vi "compileAndRunScript.vi"(6 "data":variant, 8 "error in (no error)":errorcluster, 9 "CompiledList":refnum<class "CompiledList.lvclass">, 10 "HWControllerEvents in":refnum<class "HWControllerEvents.lvclass">, 11 "Compiler in":refnum<class "Compiler.lvclass">) -> (0 "error out":errorcluster, 3 "Compiler out":refnum<class "Compiler.lvclass">)   [LabVIEW 2011, in "Compiler.lvlib" / "Compiler.lvclass"]
uses:
  Compiler.lvclass
  CompiledList/CompiledList.lvclass
  Hal/HWController/HWControllerEvents/HWControllerEvents.lvclass
  Compiler.lvclass/Compiler.ctl
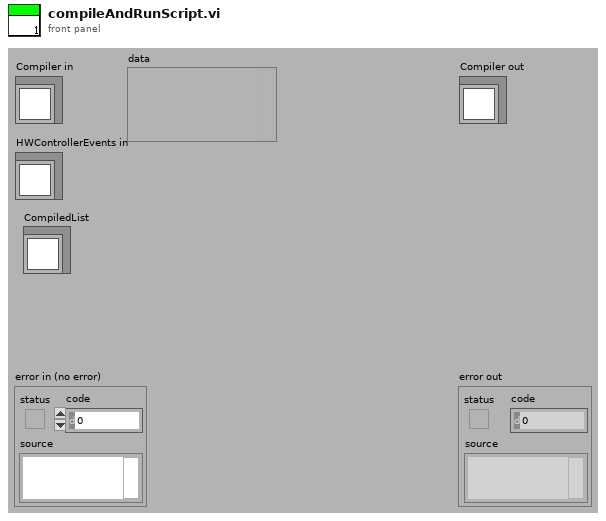
[diagram p1: front panel]
types:
  T1 = enum16{"start", "stop", "statusInquiry", "configure", "resetError", "resourcesInquiry", "reserveResources", "initialise", "resetAllChannels", "staticUpdate", "close", "HWStatus", "error", "resourcesAvailable", "resourcesReserved", "compilerError", "compiledScript", "compilingScript", "runScript", "configureCompiledScript"}
  T2 = cluster{"incomingEventTypes":cluster{"start":cluster{"Boolean":bool}, "stop":cluster{"Boolean":bool}, "statusInquiry":cluster{"Boolean":bool}, "configure":cluster{"DPScriptPath":path, "TimeStamp":string, "HWLoop?":bool}, "resetError":cluster{"Boolean":bool}, "resourcesInquiry":cluster{"Boolean":bool}, "reserveResources":cluster{"HWList":string[]}, "initialise":cluster{"HWList":string[]}, "close":cluster{"Boolean":bool}, "resetAllChannels":cluster{"Boolean":bool}, "staticChannelUpdate":cluster{"channel_address":string, "calibratedValue":dbl}, "runScript":cluster{"DPScriptPath":path, "TimeStamp":string, "HWLoop?":bool}, "compilingScript":cluster{"Path":path}, "compiledScript":cluster{"Path":path, "timeCompileAt":string}, "compilerError":cluster{"Path":path}, "configureCompiledScript":cluster{"DPScriptPath":path, "TimeStamp":string, "HWLoop?":bool, "CompiledScript":cluster{"ScriptListCompiler.lvclass":refnum<class "ScriptListCompiler.lvclass">, "aoChannels":refnum<class "AnalogOutput.lvclass">[], "doChannels":refnum<class "DigitalOutput.lvclass">[], "rfChannels":refnum<class "DDSOutput.lvclass">[]}}, "restartCompiler":cluster{"restart":bool}, "staticRfChannelUpdate":cluster{"channel_address":string, "Output":cluster{"Frequency(MHz)":dbl, "Amplitude":dbl, "Phase":dbl, "OutputForm":enum16{"Sine", "Square", "Triangle", "Arbitrary"}}}, "cameraUpdate":cluster{"Camera":string, "Type":string, "settings":path}}, "outgoingEventTypes":cluster{"HWStatus":cluster{"status":enum16{"Ready", "Compiling", "Configured", "Running", "Stopping", "Unresolved Error"}}, "error":cluster{"error out":errorcluster}, "resourcesAvailable":cluster{"availableHWList":string[], "reservedHWList":string[]}, "resourcesReserved":cluster{"reservedHWList":string[]}}}
  T3 = cluster{"DPScriptPath":path, "TimeStamp":string, "HWLoop?":bool, "CompiledScript":cluster{"ScriptListCompiler.lvclass":refnum<class "ScriptListCompiler.lvclass">, "aoChannels":refnum<class "AnalogOutput.lvclass">[], "doChannels":refnum<class "DigitalOutput.lvclass">[], "rfChannels":refnum<class "DDSOutput.lvclass">[]}}
  T4 = cluster{"DPScriptPath":path, "TimeStamp":string, "HWLoop?":bool}
  T5 = cluster{"ScriptListCompiler.lvclass":refnum<class "ScriptListCompiler.lvclass">, "aoChannels":refnum<class "AnalogOutput.lvclass">[], "doChannels":refnum<class "DigitalOutput.lvclass">[], "rfChannels":refnum<class "DDSOutput.lvclass">[]}
  T6 = cluster{"eventId":enum16{"start", "stop", "statusInquiry", "configure", "resetError", "resourcesInquiry", "reserveResources", "initialise", "resetAllChannels", "staticUpdate", "close", "HWStatus", "error", "resourcesAvailable", "resourcesReserved", "compilerError", "compiledScript", "compilingScript", "runScript", "configureCompiledScript"}, "configureCompiledScript":cluster{"DPScriptPath":path, "TimeStamp":string, "HWLoop?":bool, "CompiledScript":cluster{"ScriptListCompiler.lvclass":refnum<class "ScriptListCompiler.lvclass">, "aoChannels":refnum<class "AnalogOutput.lvclass">[], "doChannels":refnum<class "DigitalOutput.lvclass">[], "rfChannels":refnum<class "DDSOutput.lvclass">[]}}}
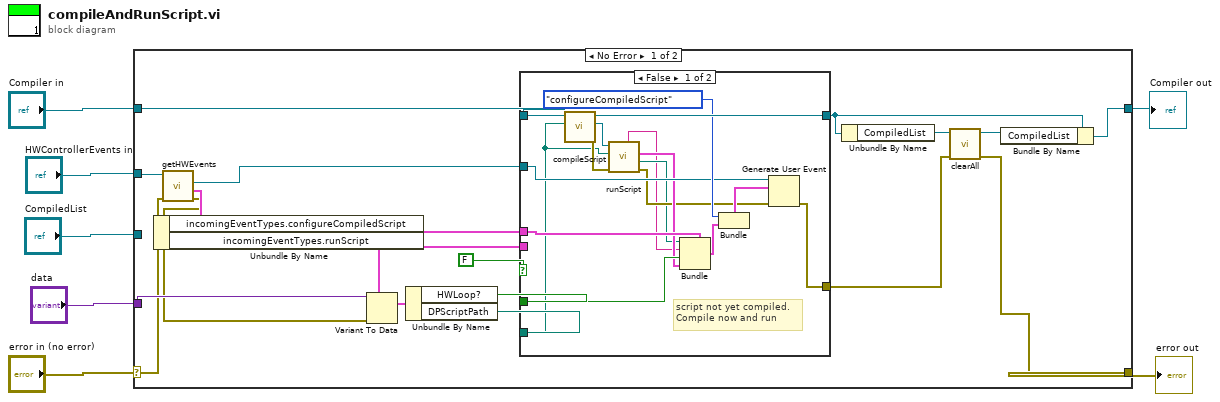
[diagram p0: block diagram]
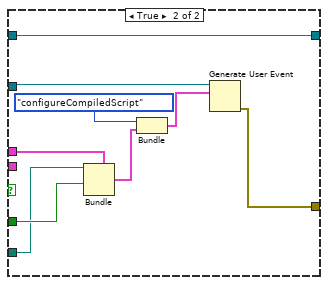
[diagram p2: hidden frame]
diagram:
  n1 = case shown="No Error" "error in (no error)" {
    selector: "error in (no error)" -> [w18 w53]
    tunnel: [w8 w53] -> w1
    tunnel: [w11 w52] -> w2
    tunnel: "Compiler in" -> [w16 w52]
    tunnel: "HWControllerEvents in" -> [w26 _]
    tunnel: "CompiledList" -> [_ _]
    tunnel: "data" -> [w24 _]
    frame No Error {
      n2 = call-dynamic "getHWEvents.vi"("error in (no error)"=w18, "HWControllerEvents in"=w26) -> ("error out"=w17:errorcluster, "eventDataTypes"=w25:T2, "HWCEvent"=w21:refnum<user-event>)  [unwired: 6 in, 1 out]
      n3 = Unbundle By Name(w25) -> ("incomingEventTypes.configureCompiledScript"=w20:T3, "incomingEventTypes.runScript"=w19:T4)
      n4 = Variant To Data(error in=w17, type=w19, Variant=w24) -> (data=w23:T4)  [unwired: 1 out]
      n5 = Unbundle By Name(w23) -> ("HWLoop?"=w22:bool, "DPScriptPath"=w15:path)
      n6 = case shown="False" FALSE {
        tunnel: [w41 w51] -> w12
        tunnel: w16 -> [w42 w51]
        tunnel: w22 -> [w36 w49]
        tunnel: w21 -> [w34 w48]
        tunnel: [w35 w44] -> w9
        tunnel: w20 -> [w37 w50]
        tunnel: w15 -> [w27 w43]
        tunnel: w19 -> [_ _]
        frame False {
          # "script not yet compiled.\nCompile now and run"
          n7 = call "compileScript.vi"("Path"=w27, "Compiler in"=w42) -> ("error out"=w32:errorcluster, "CompiledList"=w33:refnum<class "CompiledList.lvclass">, "Compiler out"=w41:refnum<class "Compiler.lvclass">)  [unwired: 7 in]
          n8 = call "runScript.vi"("error in (no error)"=w32, "Path"=w27, "CompiledList in"=w33) -> ("error out"=w30:errorcluster, "Path out"=w29:path, "CompiledScript"=w31:T5, "TimeStamp"=w28:string)  [unwired: 3 in, 2 out]
          n9 = Bundle(cluster=w37, "DPScriptPath"=w29, "TimeStamp"=w28, "HWLoop?"=w36, "CompiledScript"=w31) -> (w39:T3)
          n10 = Bundle("eventId"=T1."configureCompiledScript", "configureCompiledScript"=w39) -> (w38:T6)  [unwired: 1 in]
          n11 = Generate User Event(user event=w34, event data cluster=w38, error in=w30) -> (error out=w35:errorcluster)  [unwired: 1 out]
        }
        frame True {
          n12 = Bundle(cluster=w50, "DPScriptPath"=w43, "HWLoop?"=w49) -> (w46:T3)  [unwired: 2 in]
          n13 = Bundle("eventId"=T1."configureCompiledScript", "configureCompiledScript"=w46) -> (w45:T6)  [unwired: 1 in]
          n14 = Generate User Event(user event=w48, event data cluster=w45) -> (error out=w44:errorcluster)  [unwired: 1 in, 1 out]
        }
      }
      n15 = Unbundle By Name(w12) -> ("CompiledList"=w13:refnum<class "CompiledList.lvclass">)
      n16 = call "clearAll.vi"("error in (no error)"=w9, "CompiledList in"=w13) -> ("error out"=w8:errorcluster, "CompiledList out"=w10:refnum<class "CompiledList.lvclass">)  [unwired: 8 in]
      n17 = Bundle By Name(cluster=w12, "CompiledList"=w10) -> (w11:refnum<class "Compiler.lvclass">)
    }
    frame Error {
    }
  }
  "error out" <- w1
  "Compiler out" <- w2
